vi "data_to_xml.vi"(8 "error in (no error)":errorcluster, 11 "Experiment in":refnum<class "Experiment.lvclass">) -> (0 "error out":errorcluster, 2 "data string":string, 3 "Experiment out":refnum<class "Experiment.lvclass">)   [LabVIEW 2014, in "Experiment.lvclass"]
uses:
  Experiment.lvclass
  Experiment.lvclass/Experiment.ctl
  Globals.vi
  Camera/Hamamatsu_C9100-13/Hamamatsu_C9100-13.lvclass
  Counter/Counter.lvclass
  TTL_input/TTL_input.lvclass
  Analog_Input/Analog_Input.lvclass
  Camera/Camera.lvclass
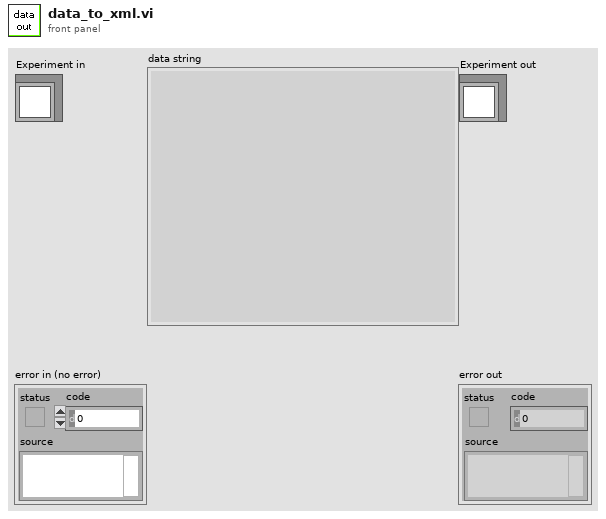
[diagram p1: front panel]
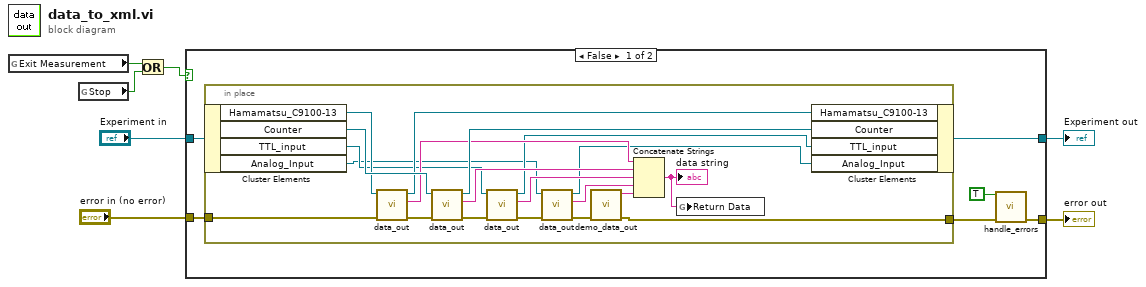
[diagram p0: block diagram]
diagram:
  n1 = global read "Globals.vi" "Exit Measurement"() -> (w4:bool)
  n2 = global read "Globals.vi" "Stop"() -> (w3:bool)
  n3 = Or(x=w4, y=w3) -> (x .or. y?=w2:bool)
  n4 = case shown="False" w2 {
    tunnel: [w12 w35] -> w6
    tunnel: "Experiment in" -> [w13 w35]
    tunnel: [w10 w34] -> w5
    tunnel: "error in (no error)" -> [w8 w34]
    frame False {
      n5 = in-place {
        in-place-border: [w21] -> w11
        in-place-border: w8 -> [w28]
        n6 = in-place-cluster #1(w13) -> ("Hamamatsu_C9100-13"=w31:refnum<class "Hamamatsu_C9100-13.lvclass">, "Counter"=w33:refnum<class "Counter.lvclass">, "TTL_input"=w25:refnum<class "TTL_input.lvclass">, "Analog_Input"=w17:refnum<class "Analog_Input.lvclass">)
        n7 = call-dynamic "data_out.vi"("error in (no error)"=w28, "Hamamatsu_C9100-13 in"=w31) -> ("error out"=w29:errorcluster, "camera data string"=w27:string, "Hamamatsu_C9100-13 out"=w30:refnum<class "Hamamatsu_C9100-13.lvclass">)  [unwired: 7 in]
        n8 = call-dynamic "data_out.vi"("error in (no error)"=w29, "Counter in"=w33) -> ("error out"=w23:errorcluster, "counter data string"=w26:string, "Counter out"=w32:refnum<class "Counter.lvclass">)  [unwired: 7 in]
        n9 = call-dynamic "data_out.vi"("error in (no error)"=w23, "TTL_input in"=w25) -> ("error out"=w19:errorcluster, "TTL data string"=w22:string, "TTL_input out"=w24:refnum<class "TTL_input.lvclass">)  [unwired: 7 in]
        n10 = call-dynamic "data_out.vi"("error in (no error)"=w19, "Analog_Input (in)"=w17) -> ("error out"=w18:errorcluster, "AI data string"=w15:string, "Analog_Input"=w16:refnum<class "Analog_Input.lvclass">)  [unwired: 7 in]
        n11 = call "demo_data_out.vi"("error in (no error)"=w18) -> ("error out"=w21:errorcluster, "camera data string"=w14:string)  [unwired: 9 in]
        n12 = Concatenate Strings(w27, w26, w22, w15, w14) -> (w20:string)
        "data string" <- w20
        n13 = global write "Globals.vi" "Return Data"(w20) -> ()
        n14 = in-place-cluster #1("Hamamatsu_C9100-13"=w30, "Counter"=w32, "TTL_input"=w24, "Analog_Input"=w16) -> (w12:refnum<class "Experiment.lvclass">)
      }
      n15 = call "handle_errors.vi"("Exit Operation"=TRUE ("Exit Measurement"), "error in (no error)"=w11) -> ("error out"=w10:errorcluster)  [unwired: 13 in]
    }
    frame True {
    }
  }
  "error out" <- w5
  "Experiment out" <- w6
